vi "Parametric Sweep.vi"() -> ()   [LabVIEW 2013]
uses:
  Power Supply.lvlib
  Fixture.lvlib
  Oscilloscope.lvlib
panel:
  in  "serial number":string="1"
  out "Intensity Graph":dbl[][](graph)
  in  "Channel":i32=1
  out "error out":errorcluster
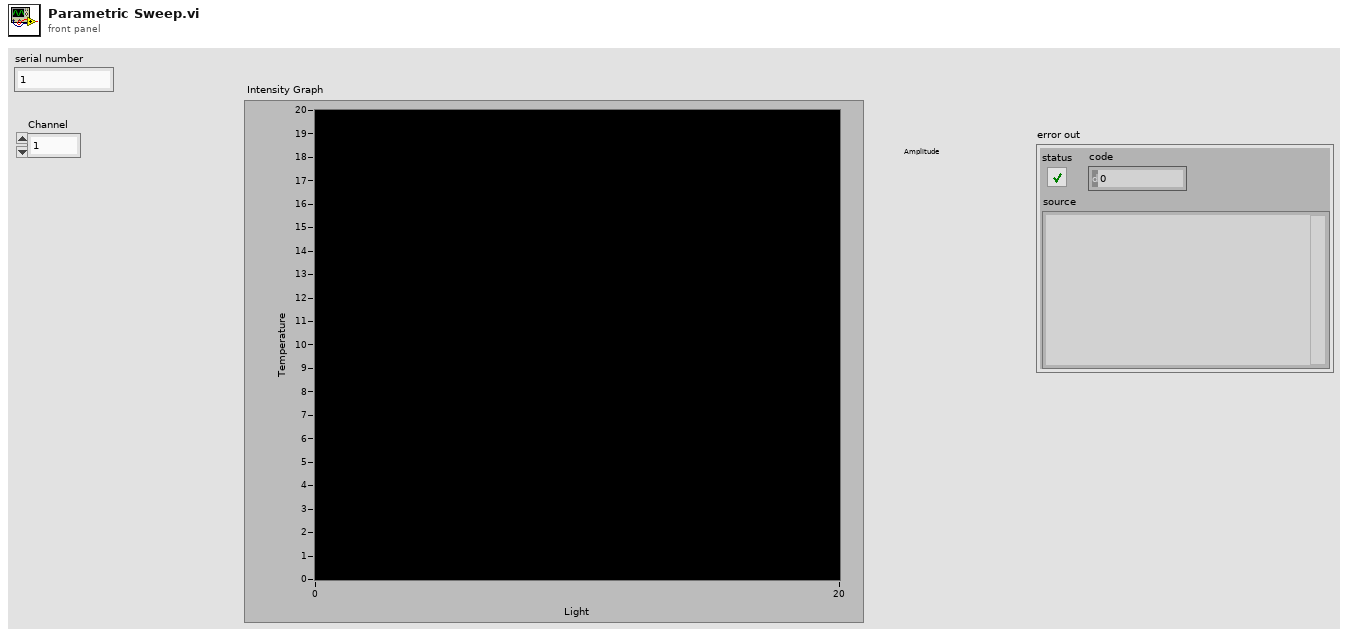
[diagram p1: front panel]
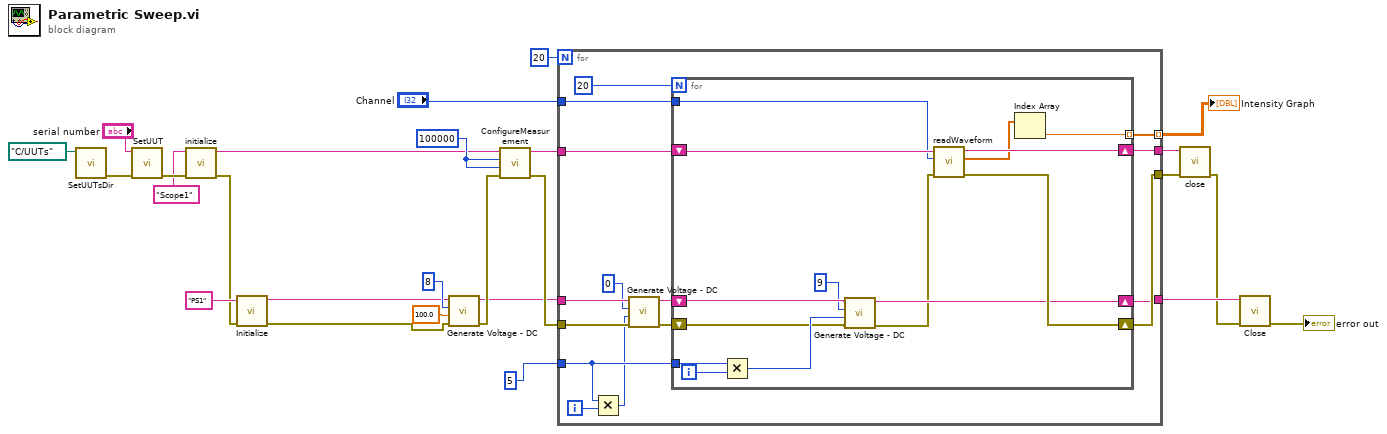
[diagram p0: block diagram]
diagram:
  w12 = 100000 ("numSamples")
  n1 = call "SetUUTsDir.vi"("UUTDirectory"=path "C:/UUTs") -> ("error out"=w26:errorcluster)  [unwired: 10 in]
  n2 = call "SetUUT.vi"("error in (no error)"=w26, "Serial Number"="serial number") -> ("error out"=w16:errorcluster)  [unwired: 9 in]
  n3 = call "initialize.vi"("error in (no error)"=w16, "Scope in"="Scope1" ("Resource Name")) -> ("error out"=w17:errorcluster, "Scope out"=w11:string)  [unwired: 8 in]
  n4 = call "Initialize.vi"("error in (no error)"=w17, "Power Supply in"="PS1" ("Resource Name")) -> ("error out"=w1:errorcluster, "Power Supply out"=w2:string)  [unwired: 8 in]
  n5 = call "Generate Voltage - DC.vi"("error in (no error)"=w1, "Output Voltage"=100.0 ("outputVoltage"), "Channel"=8 ("channel"), "Power Supply in"=w2) -> ("error out"=w6:errorcluster, "Power Supply out"=w3:string)  [unwired: 6 in]
  n6 = call "ConfigureMeasurement.vi"("error in (no error)"=w6, "Samples Per Second"=w12, "Number of Samples"=w12, "Scope in"=w11) -> ("error out"=w14:errorcluster, "Scope out"=w13:string)  [unwired: 6 in]
  n7 = for {
    N: 20 -> [_]
    tunnel: [w38] -> w25
    tunnel: [w41] -> w20
    tunnel: [w40] -> w18
    tunnel: w14 -> [w30]
    tunnel: w13 -> [w39]
    tunnel: "Channel" -> [w37]
    tunnel: [w36] -> w9 mode=indexing
    tunnel: 5 ("numSamples") -> [w33]
    tunnel: w3 -> [w29]
    i -> [w34]
    n8 = Multiply(x=w33, y=w34) -> (x*y=w27:i32)
    n9 = call "Generate Voltage - DC.vi"("error in (no error)"=w30, "Output Voltage"=w27, "Channel"=0 ("channel"), "Power Supply in"=w29) -> ("error out"=w32:errorcluster, "Power Supply out"=w31:string)  [unwired: 6 in]
    n10 = for {
      N: 20 -> [_]
      tunnel: w37 -> [w52]
      shift-right: [w49] -> w38
      shift-left: w31 -> [w43]
      shift-right: [w54] -> w40
      shift-left: w39 -> [w53]
      tunnel: [w50] -> w36 mode=indexing
      shift-right: [w55] -> w41
      shift-left: w32 -> [w44]
      tunnel: w33 -> [w45]
      i -> [w47]
      n11 = Multiply(x=w45, y=w47) -> (x*y=w46:i32)
      n12 = call "Generate Voltage - DC.vi"("error in (no error)"=w44, "Output Voltage"=w46, "Channel"=9 ("channel"), "Power Supply in"=w43) -> ("error out"=w48:errorcluster, "Power Supply out"=w49:string)  [unwired: 6 in]
      n13 = call "readWaveform.vi"("error in (no error)"=w48, "Channel"=w52, "Scope in"=w53) -> ("error out"=w55:errorcluster, "Result"=w51:dbl[], "Scope out"=w54:string)  [unwired: 6 in]
      n14 = Index Array(array=w51) -> (element=w50:dbl)  [unwired: 1 in]
    }
  }
  "Intensity Graph" <- w9
  n15 = call "close.vi"("error in (no error)"=w20, "Scope in"=w18) -> ("error out"=w19:errorcluster)  [unwired: 9 in]
  n16 = call "Close.vi"("error in (no error)"=w19, "Power Supply in"=w25) -> ("error out"=→"error out":errorcluster)  [unwired: 9 in]
